vi "Process Player Movement Inputs.vi"(11 "Ship in":refnum<class "Ship.lvclass">) -> (3 "Ship out":refnum<class "Ship.lvclass">)   [LabVIEW 2021, in "Ship.lvclass"]
uses:
  Ship.lvclass
  Ship.lvclass/Ship.ctl
  Control State/Control State.lvclass
  Element/Element.lvclass
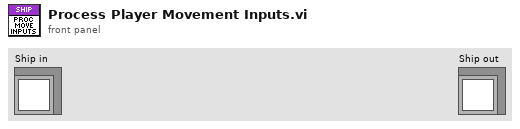
[diagram p1: front panel]
types:
  T1 = typedef "Control State.lvclass/Button State.ctl" = enum16{"Undefined", "Pressed", "Released", "Held", "Not Held"}
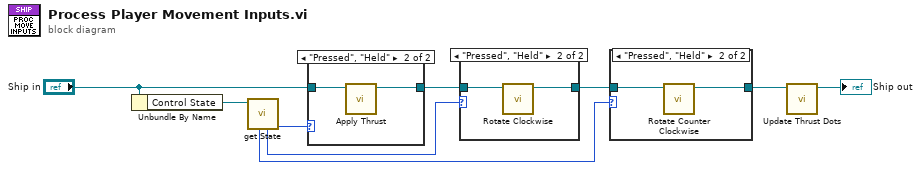
[diagram p0: block diagram]
diagram:
  n1 = Unbundle By Name("Ship in") -> ("Control State"=w3:refnum<class "Control State.lvclass">)
  n2 = call "get State.vi"("Control State in"=w3) -> ("Thrust"=w5:T1, "Rotate Clockwise"=w6:T1, "Rotate Counter Clockwise"=w9:T1)  [unwired: 6 in, 2 out]
  n3 = case shown="\"Pressed\", \"Held\"" w5 {
    tunnel: "Ship in" -> [w10 w12]
    tunnel: [w10 w11] -> w7
    frame Default {
    }
    frame "Pressed", "Held" {
      n4 = call "Apply Thrust.vi"("Element in"=w12) -> ("Element out"=w11:refnum<class "Ship.lvclass">)  [unwired: 10 in]
    }
  }
  n5 = case shown="\"Pressed\", \"Held\"" w6 {
    tunnel: w7 -> [w13 w15]
    tunnel: [w13 w14] -> w8
    frame Default {
    }
    frame "Pressed", "Held" {
      n6 = call "Rotate Clockwise.vi"("Element in"=w15) -> ("Element out"=w14:refnum<class "Ship.lvclass">)  [unwired: 10 in]
    }
  }
  n7 = case shown="\"Pressed\", \"Held\"" w9 {
    tunnel: w8 -> [w16 w18]
    tunnel: [w16 w17] -> w1
    frame Default {
    }
    frame "Pressed", "Held" {
      n8 = call "Rotate Counter Clockwise.vi"("Element in"=w18) -> ("Element out"=w17:refnum<class "Ship.lvclass">)  [unwired: 10 in]
    }
  }
  n9 = call "Update Thrust Dots.vi"("Ship in"=w1) -> ("Ship out"=→"Ship out":refnum<class "Ship.lvclass">)  [unwired: 10 in]
